vi "Configure Parameter.vi"(8 "error in (no error)":errorcluster, 10 "Configure Parameter":T1={"Temp Parameter"={"Temperature setpoint"=40.0, "upper limit"=80.0, "lower limit"=0.0}, "Humidity Parameter"={"Humidity setpoint"=50.0, "upper limit"=80.0, "lower limit"=0.0}}, 11 "ARS-0220 in":refnum<class "ARS-0220.lvclass">) -> (0 "error out":errorcluster, 3 "ARS-0220 out":refnum<class "ARS-0220.lvclass">)   [LabVIEW 2021, in "Environment Chamber.lvlib" / "ARS-0220.lvclass"]
uses:
  ARS-0220.lvclass
  Configure Parameter.ctl
  ARS-0220.lvclass/ARS-0220.ctl
  Support Libraries/Climatic Chamber/Climatic Chamber.lvlib
  Environment Chamber.lvlib
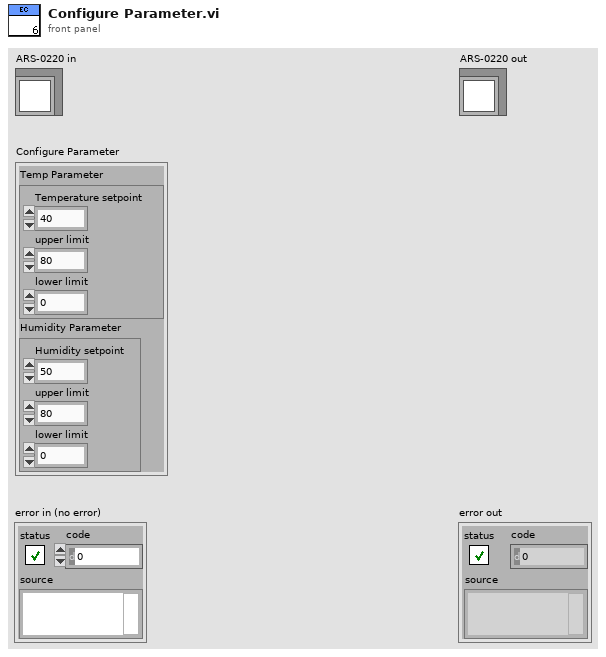
[diagram p1: front panel]
types:
  T1 = typedef "Environment Chamber.lvlib/Configure Parameter.ctl" = cluster{"Temp Parameter":cluster{"Temperature setpoint":dbl, "upper limit":dbl, "lower limit":dbl}, "Humidity Parameter":cluster{"Humidity setpoint":dbl, "upper limit":dbl, "lower limit":dbl}}
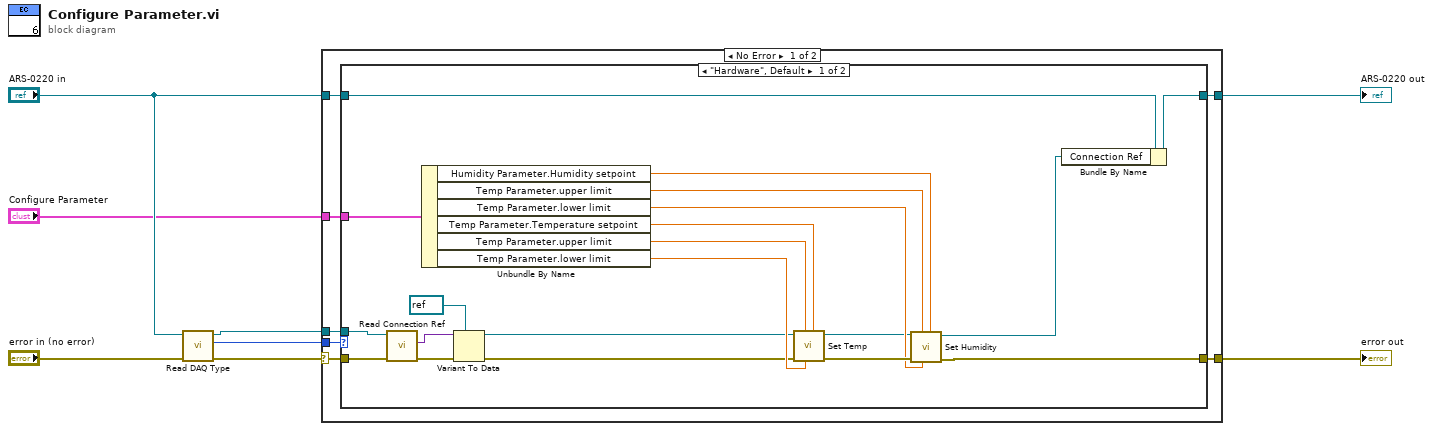
[diagram p0: block diagram]
diagram:
  n1 = call "Read DAQ Type.vi"("error in (no error)"="error in (no error)", "ARS-0220 in"="ARS-0220 in") -> ("error out"=w6:errorcluster, "DAQ Type"=w4:enum16{"Hardware", "Simulation"}, "ARS-0220 out"=w2:refnum<class "ARS-0220.lvclass">)  [unwired: 7 in]
  n2 = case shown="No Error" w6 {
    selector: w6 -> [w12 w38]
    tunnel: "ARS-0220 in" -> [w15 w39]
    tunnel: [w14 w39] -> w7
    tunnel: w4 -> [w13 _]
    tunnel: [w9 w38] -> w3
    tunnel: "Configure Parameter" -> [w11 _]
    tunnel: w2 -> [w10 _]
    frame No Error {
      n3 = case shown="\"Hardware\", Default" w13 {
        tunnel: w15 -> [w35 w37]
        tunnel: [w18 w37] -> w14
        tunnel: w12 -> [w33 w36]
        tunnel: w11 -> [w34 _]
        tunnel: w10 -> [w24 _]
        tunnel: [w16 w36] -> w9
        frame "Hardware", Default {
          n4 = call "Read Connection Ref.vi"("error in (no error)"=w33, "ARS-0220 in"=w24) -> ("error out"=w25:errorcluster, "Connection Ref"=w22:variant)  [unwired: 7 in, 1 out]
          n5 = Unbundle By Name(w34) -> ("Humidity Parameter.Humidity setpoint"=w28:dbl, "Temp Parameter.upper limit"=w27:dbl, "Temp Parameter.lower limit"=w26:dbl, "Temp Parameter.Temperature setpoint"=w32:dbl, "Temp Parameter.upper limit"=w31:dbl, "Temp Parameter.lower limit"=w30:dbl)
          n6 = Variant To Data(error in=w25, type=refnum<visa-resource-name> refnum ("VISA resource name"), Variant=w22) -> (data=w20:refnum<visa-resource-name>, error out=w23:errorcluster)
          n7 = call "Set Temp.vi"("Temp"=w32, "Lower Limit"=w30, "Upper Limit"=w31, "error in (no error)"=w23, "VISA resource name"=w20) -> ("error out"=w29:errorcluster, "VISA resource name out"=w19:refnum<visa-resource-name>)  [unwired: 5 in]
          n8 = call "Set Humidity.vi"("Humidity"=w28, "Lower Limit"=w26, "Upper Limit"=w27, "error in (no error)"=w29, "VISA resource name"=w19) -> ("error out"=w16:errorcluster, "VISA resource name out"=w17:refnum<visa-resource-name>)  [unwired: 5 in]
          n9 = Bundle By Name(cluster=w35, "Connection Ref"=w17) -> (w18:refnum<class "ARS-0220.lvclass">)
        }
        frame "Simulation" {
        }
      }
    }
    frame Error {
    }
  }
  "error out" <- w3
  "ARS-0220 out" <- w7
